vi "Exemple_Model_Selection_Train_Test_Split.vi"() -> ()   [LabVIEW 2020]
panel:
  out "Y_Train":T1
  out "Y_Test":T1
  out "X_Train":T1
  out "X_Test":T1
  in  "Y":string[][](array[string])=[["0"], ["1"], ["2"], ["3"], ["4"]]
  in  "X":string[][](array[string])=[["0", "1"], ["2", "3"], ["4", "5"], ["6", "7"], ["8", "9"]]
  out "error out":errorcluster caption="sortie d'erreur"
  in  "error in (no error)":errorcluster caption="entrée d'erreur (pas d'erreur)"
  in  "TestTrain":T2={"test_size"=-1.0, "train_size"=-1.0, "random_state"=-1, "shuffle"=TRUE, "stratify"=[]} {"random_state" min=-1; "train_size" min=-1.0; "test_size" min=-1.0}
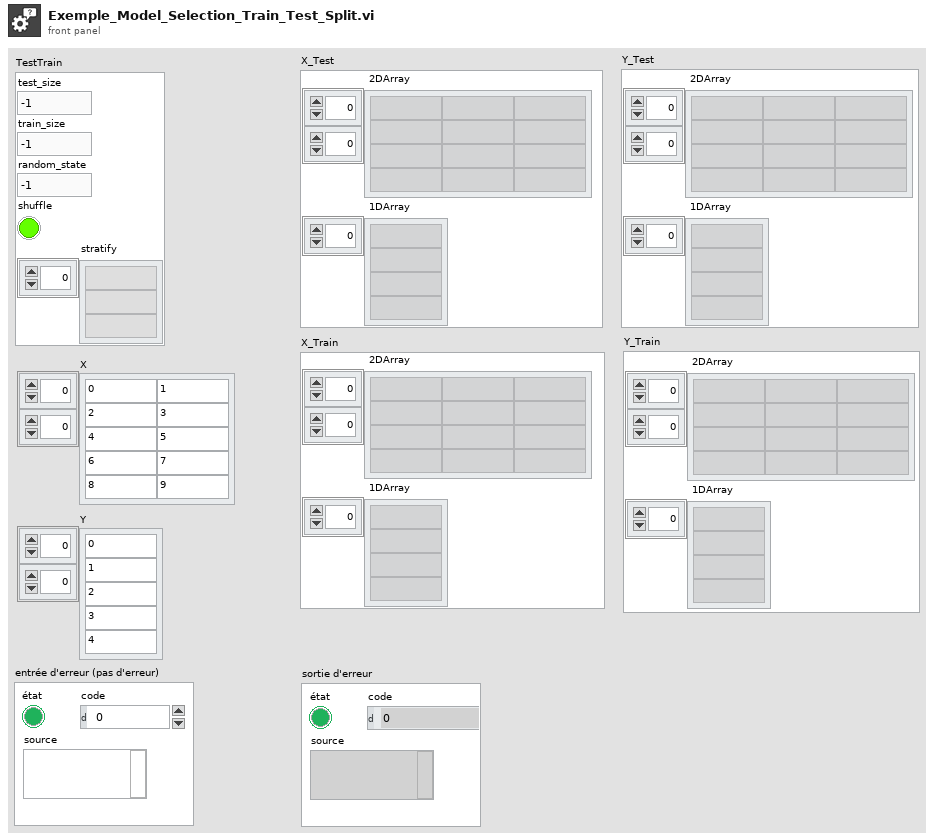
[diagram p1: front panel]
types:
  T1 = cluster{" 4DArray":cluster{"1":string[][], "2":string[][]}[], " 3DArray":cluster{"Tableau":string[][]}[], "Sparse Matrix 2DArray":string[][], " 2DArray":string[][], " 1DArray":string[]}
  T2 = cluster{"test_size":dbl, "train_size":dbl, "random_state":i32, "shuffle":bool, "stratify":string[]}
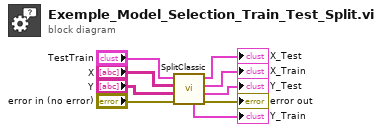
[diagram p0: block diagram]
diagram:
  n1 = call "SplitClassic.vi"("error in (no error)"="error in (no error)", "Y"="Y", "X"="X", "TestTrain"="TestTrain") -> ("error out"=→"error out":errorcluster, "Y_Test"=→"Y_Test":T1, "X_Train"=→"X_Train":T1, "X_Test"=→"X_Test":T1, "Y_Train"=→"Y_Train":T1)  [unwired: 3 in]
